vi "Shutdown.vi"(8 "error in":errorcluster, 11 "Instruments in":refnum<class "Instruments.lvclass">) -> (0 "error out":errorcluster, 3 "Instruments out":refnum<class "Instruments.lvclass">)   [LabVIEW 2023, in "Instruments.lvlib" / "Instruments.lvclass"]
uses:
  Library/Instruments.lvclass
  C:/Users/Public/Documents/Development/builds/Engine/Engine.lvlibp/Project/Engine.lvclass
  C:/Users/Public/Documents/Development/builds/Engine/Actor Framework.lvlibp/1abvi3w/vi.lib/ActorFramework/Actor/Actor.lvclass
  builds/Engine/Engine.lvlibp/Accessors/Read Report Queue.vi
  builds/Engine/Actor Framework.lvlibp/1abvi3w/vi.lib/ActorFramework/Actor/Read Actor Label.vi
  builds/Tools/QDMH.lvlibp/Private/Enqueue Bundled Element.vi
  builds/Tools/QDMH.lvlibp/QDMH.lvclass
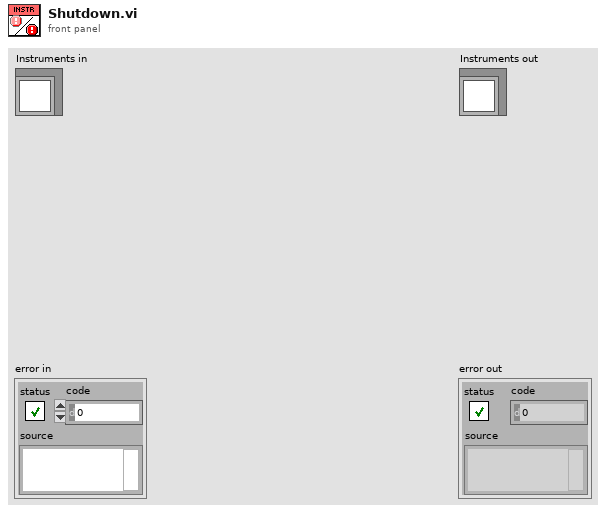
[diagram p1: front panel]
types:
  T1 = cluster{"Accessors:Actor Label":string, string[], variant[]}
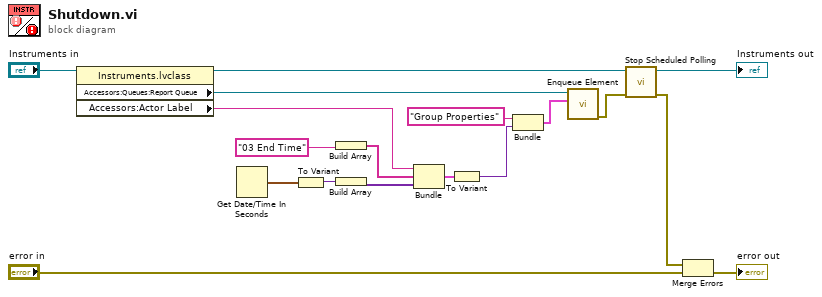
[diagram p0: block diagram]
diagram:
  n1 = property class="Instruments.lvclass"(reference="Instruments in") -> (reference out=w4:refnum<class "Instruments.lvclass">, "Accessors:Queues:Report Queue"=w5:refnum<class "QDMH.lvclass">, "Accessors:Actor Label"=w15:string)  [unwired: 1 in, 1 out]
  n2 = Get Date/Time In Seconds() -> (seconds since 1Jan1904=w9:timestamp)
  n3 = To Variant(anything=w9) -> (Variant=w10:variant)
  n4 = Build Array("03 End Time") -> (w14:string[])
  n5 = Build Array(w10) -> (w13:variant[])
  n6 = Bundle("Accessors:Actor Label"=w15, w14, w13) -> (w11:T1)  [unwired: 1 in]
  n7 = To Variant(anything=w11) -> (Variant=w12:variant)
  n8 = Bundle("Group Properties", "Variant"=w12) -> (w6:cluster{string, "Variant":variant})  [unwired: 1 in]
  n9 = call-poly "Enqueue Element.vi"("element"=w6, "QDMH in"=w5) -> ("error out"=w2:errorcluster)  [unwired: 8 in, 1 out]
  n10 = call "Stop Scheduled Polling.vi"("error in"=w2, "Instruments in"=w4) -> ("error out"=w1:errorcluster, "Instruments out"=→"Instruments out":refnum<class "Instruments.lvclass">)  [unwired: 8 in]
  n11 = Merge Errors(w1, "error in") -> (→"error out":errorcluster)
